vi "master_python_v3.0.vi"() -> ()   [LabVIEW 2026]
uses:
  <vilib>/Utility/error.llb/DialogType.ctl
  <vilib>/DAQmx/read.llb/DAQmx Read (Analog 1D Wfm NChan NSamp).vi
  <vilib>/DAQmx/miscellaneous.llb/DAQmx Fill In Error Info.vi
  Nanostage/Madlib.dll
  <vilib>/DAQmx/write.llb/DAQmx Write (Analog 2D DBL NChan NSamp).vi
  <vilib>/Utility/inputDevices.llb/keyboardAcquire.vi
panel:
  in  "Save Spectrum":bool
  in  "#":i32=1
  in  "Duration (s)":dbl=2.0
  out "z 2":dbl
  out "QPD":dbl
  out "Pos 0":dbl
  in  "Comment":string
  out "loop iteration":i32
  out "x start":dbl
  out "y start":dbl
  out "z start":dbl
  out "start iteration":dbl
  out "data":waveform(dbl)[](array[waveform])
  out "Numeric 2":i32
  out "Numeric":i32
  out "stop Ind":bool
  in  "Tab Control":T1(tab)
  in  "Apply Force":bool
  out "Waveform Chart 6":waveform(dbl)(graph)
  out "Waveform Chart 5":waveform(dbl)(graph)
  in  "stop":bool
  in  "Record Data":bool
  in  "New File?":bool caption="new_file"
  out "QPD Position":cluster{"Array":dbl[], "Array":dbl[]}(graph)
  out "MT channels":waveform(dbl)[](graph)
  out "QPD Precise Position":cluster{"Array":dbl[], "Array":dbl[]}(graph)
  out "QPD Sum (Volt)":waveform(dbl)(graph)
  out "x":dbl
  out "y":dbl
  out "z":dbl
  in  "<":bool
  in  ">":bool
  in  "v":bool
  in  "^":bool
  in  "Down":bool
  in  "Up":bool
  in  "Fine":dbl=50.0
  in  "Step Size (nm)":bool
  in  "Course":dbl=500.0
  in  "Enable\ntapping":bool
  in  "DELAY (ms)":u32=10
  in  "x amplitude\n(um)":dbl
  in  "speed":i32=1
  in  "z amplitude (um)":dbl
  out "# oscillations":dbl
  in  "y amplitude\n(um)":dbl min=-25.0 max=25.0 step=0.05
  in  "Samples":u16=100 min=1 step=1
  in  "Centre":bool
  in  "Power Spectrum":bool
  in  "Boolean":bool
  in  "Frequency":dbl=1.0 min=0.0 max=100.0 step=0.01
  in  "Amplitude":dbl=0.5 min=0.1 max=0.9 step=0.1
  in  "# Cycles":dbl=50.0 min=0.0 max=10000.0 step=0.001
  in  "Start Signal\nGen":bool
  in  "Desired Force (pN)":dbl step=0.01
  out "Measured Force (pN)":dbl(slide) scale=-2.0..2.0
  out "QPD nLR":waveform(dbl)(graph)
  out "QPD nBT":waveform(dbl)(graph)
  in  "Filename":path=path "C:/Users/localadmin/Desktop/220601 beadscan/7umscan2umbead.lvm"
  in  "Set 0 pN Position":bool
  out "QPD0":dbl
  in  "reinitialize?":bool
  in  "Conversion factor (pN/V)":dbl=1.0
  in  "output range":cluster{"output high":dbl, "output low":dbl}={"output high"=0.1, "output low"=-0.1} {"output low" format="%.2f"; "output high" format="%.2f"}
  in  "PID gains":T2={"proportional gain (Kc)"=0.5, "integral time (Ti, min)"=0.0, "derivative time (Td, min)"=0.0} {"derivative time (Td, min)" min=-1e-18 max=1000000000000000.0 step=1e-05 format="%.3f"; "integral time (Ti, min)" min=-1e-18 step=1e-05 format="%.6f"; "proportional gain (Kc)" min=-1e-18 step=1e-05 format="%.5f"}
  out "Setpoint":dbl
  out "PID output":dbl format="%.2f"
  # "Left= anticlockwise"
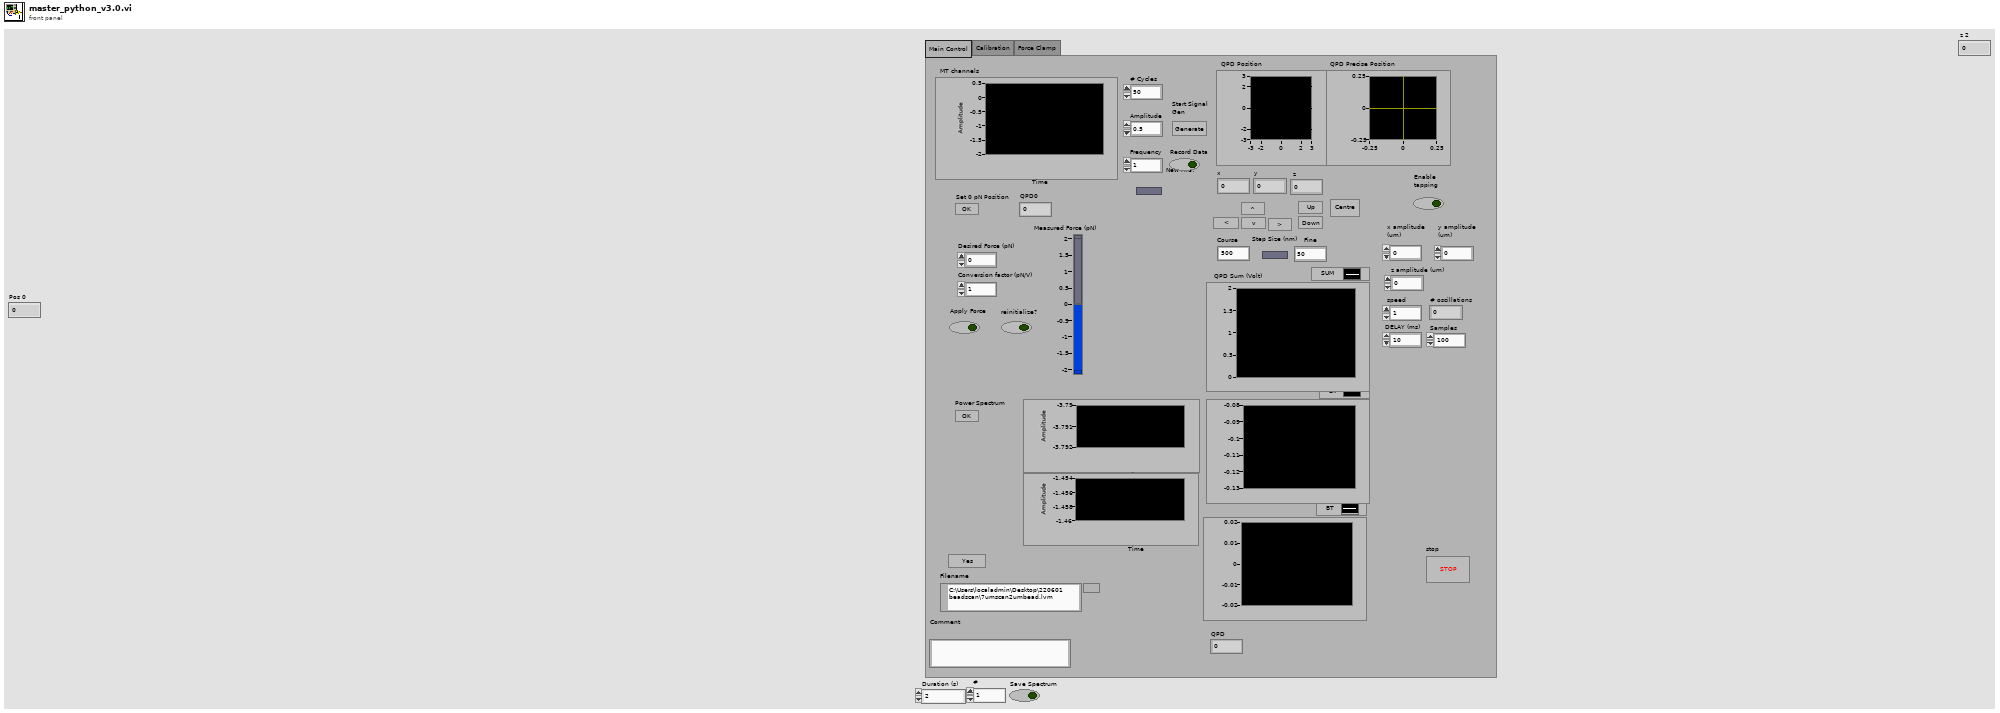
[diagram p1: front panel]
types:
  T1 = enum32{"Main Control", "Calibration", "Force Clamp"}
  T2 = cluster{"proportional gain (Kc)":dbl, "integral time (Ti, min)":dbl, "derivative time (Td, min)":dbl}
  T3 = typedef "DialogType.ctl" = u16
  T4 = enum16{"Centre", "Move", "Tapping", "Calibration"}
  T5 = cluster{"kp":dbl, "ti":dbl, "td":dbl, "index":i32, "process_variable":dbl, "derivative_action":dbl, "integrated_error":dbl, "error":dbl, "output":dbl}
  T6 = enum16{"0", "1", "2", "3", "4", "5", "6", "7", "8", "9", "A", "B", "C", "D", "E", "F", "G", "H", "I", "J", "K", "L", "M", "N", "O", "P", "Q", "R", "S", "T", "U", "V", "W", "X", "Y", "Z", "F1", "F2", "F3", "F4", "F5", "F6", "F7", "F8", "F9", "F10", "F11", "F12", "F13", "F14", "F15", "ADD", "BACK", "BACKSLASH", "CAPITAL", "COMMA", "DECIMAL", "DELETE", "DIVIDE", "DOWN", "END", "EQUALS", "ESCAPE", "GRAVE (`)", "HOME", "INSERT", "LBRACKET", "LCONTROL", "LEFT", "L ALT", "LSHIFT", "LWIN", "MINUS", "MULTIPLY", "NEXT", "NUMLOCK", "NUMPAD_0", "NUMPAD_1", "NUMPAD_2", "NUMPAD_3", "NUMPAD_4", "NUMPAD_5", "NUMPAD_6", "NUMPAD_7", "NUMPAD_8", "NUMPAD_9", "PAUSE", "PERIOD", "PRIOR (PG UP)", "RBRACKET", "RCONTROL", "RETURN", "RIGHT", "R ALT", "RSHIFT", "RWIN", "SCROLL", "SEMICOLON", "SLASH", "SPACE", "SUBTRACT", "TAB", "UP", "ENTER (num pad)", "' (quote)"}[]
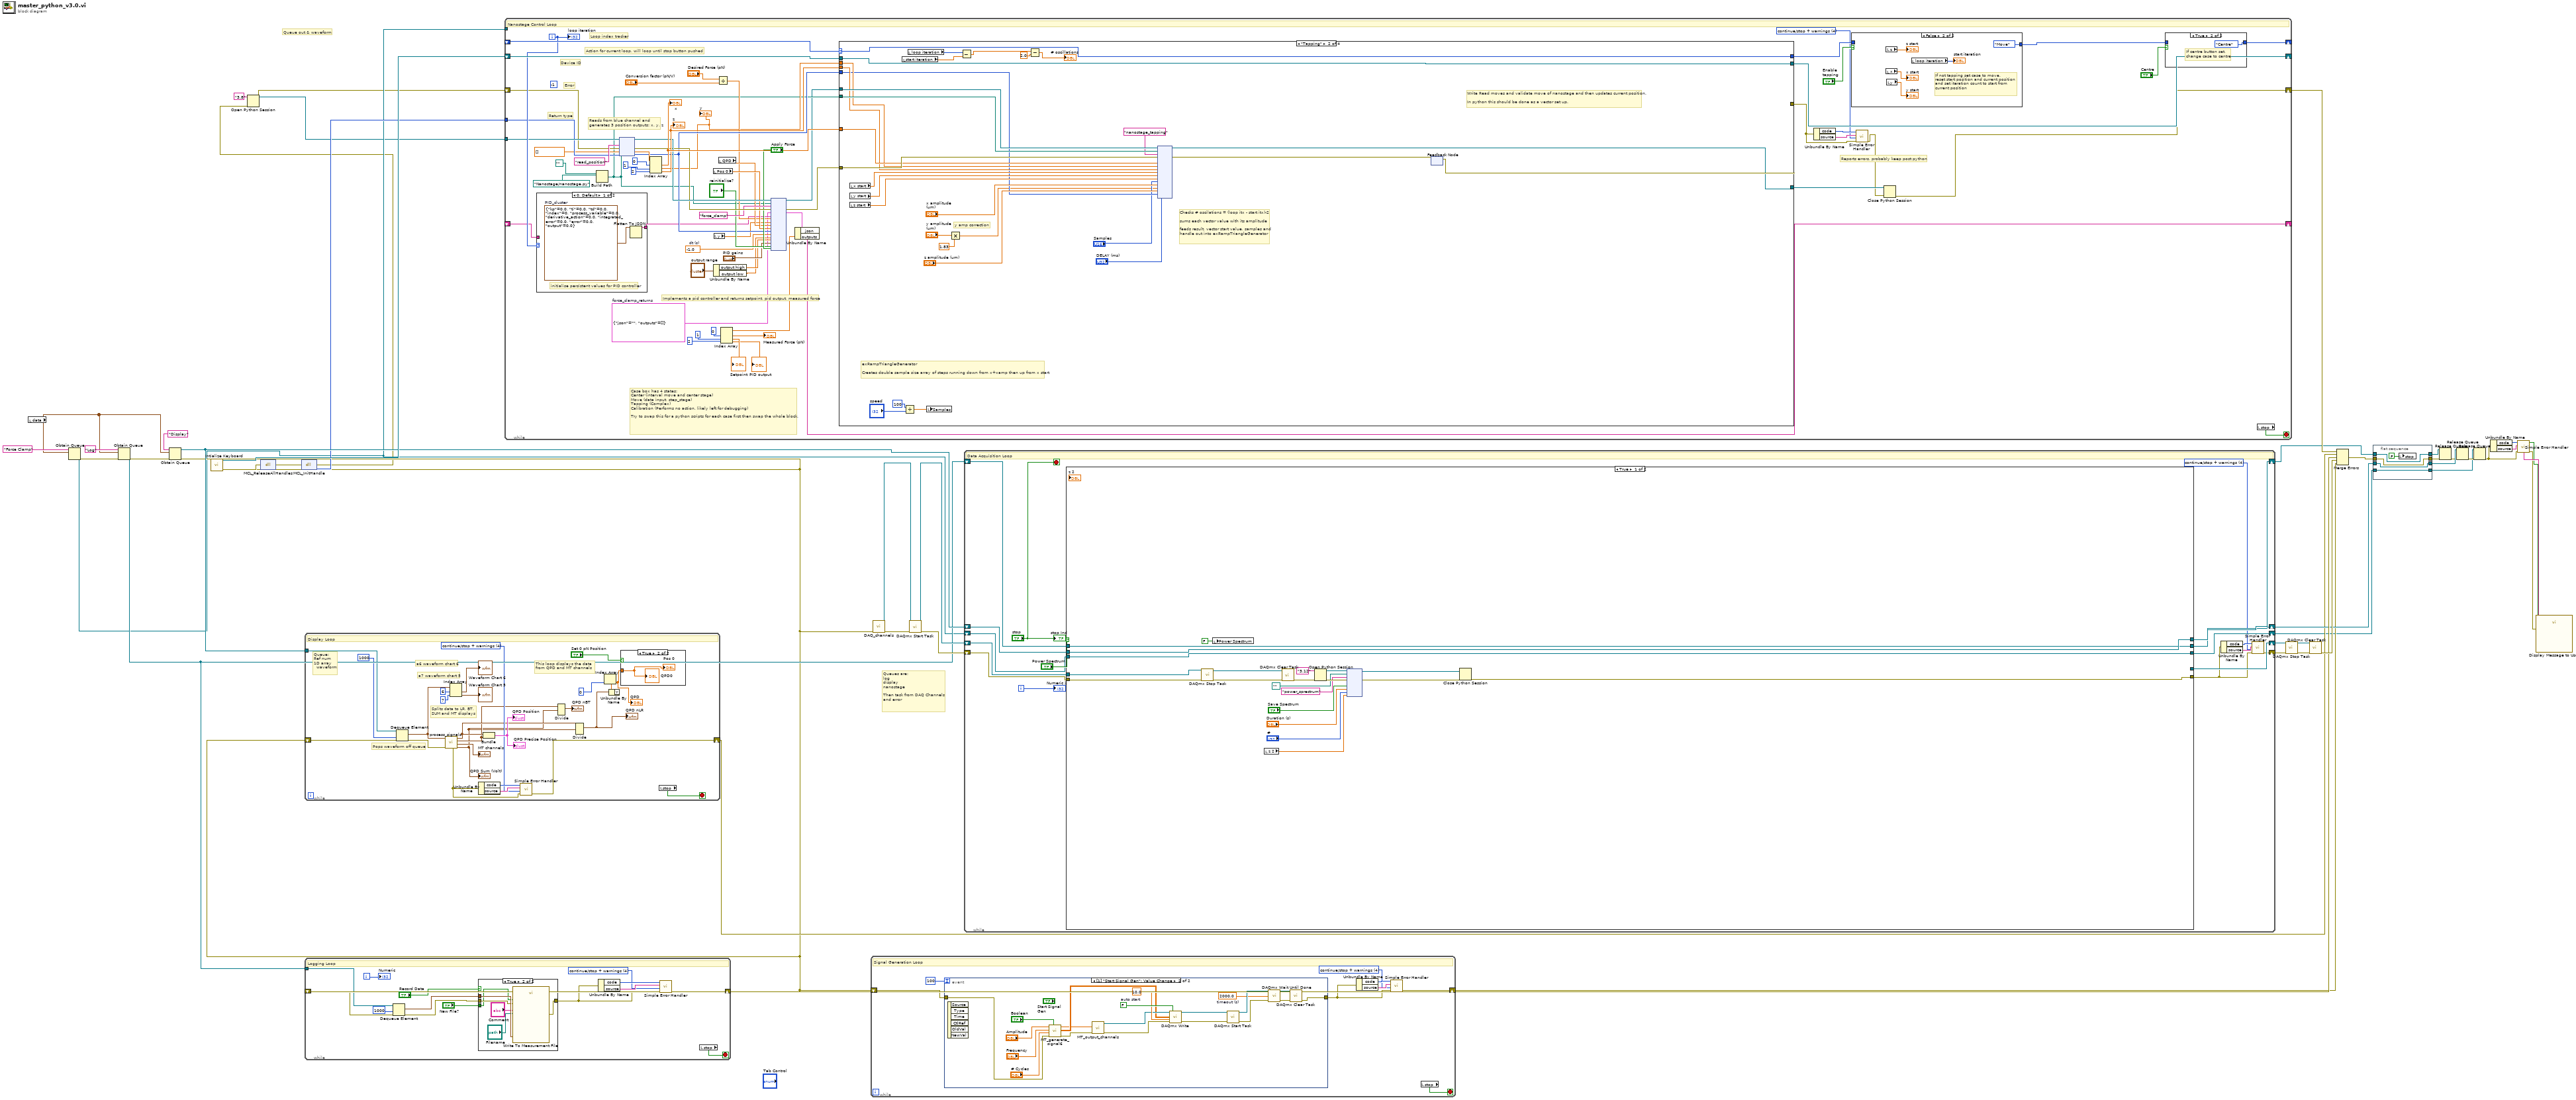
[diagram p0: block diagram]
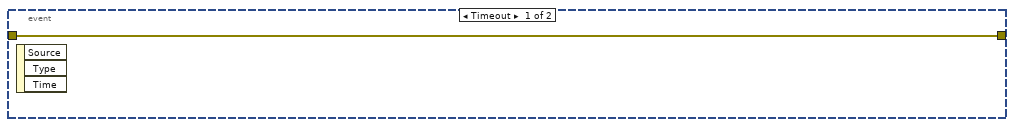
[diagram p2: hidden frame]
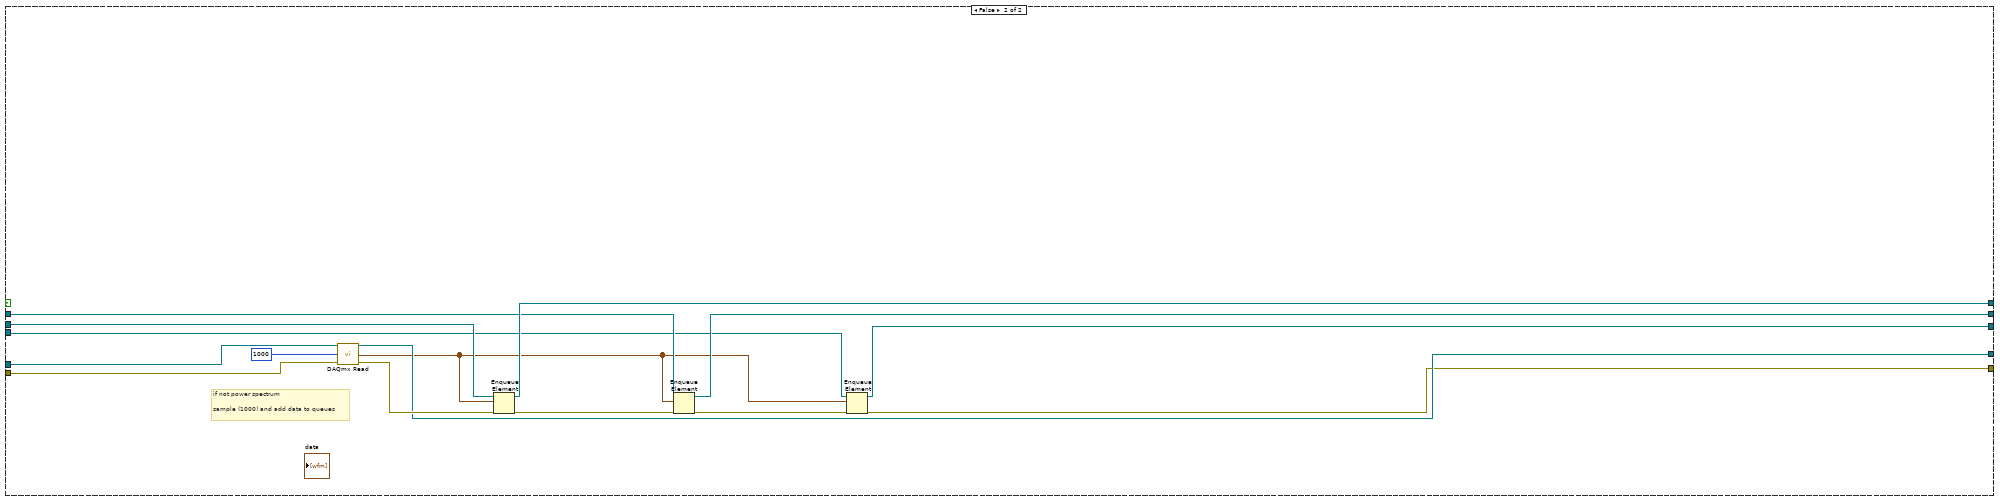
[diagram p3: hidden frame]
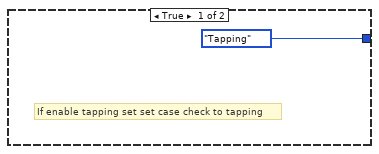
[diagram p7: hidden frame]
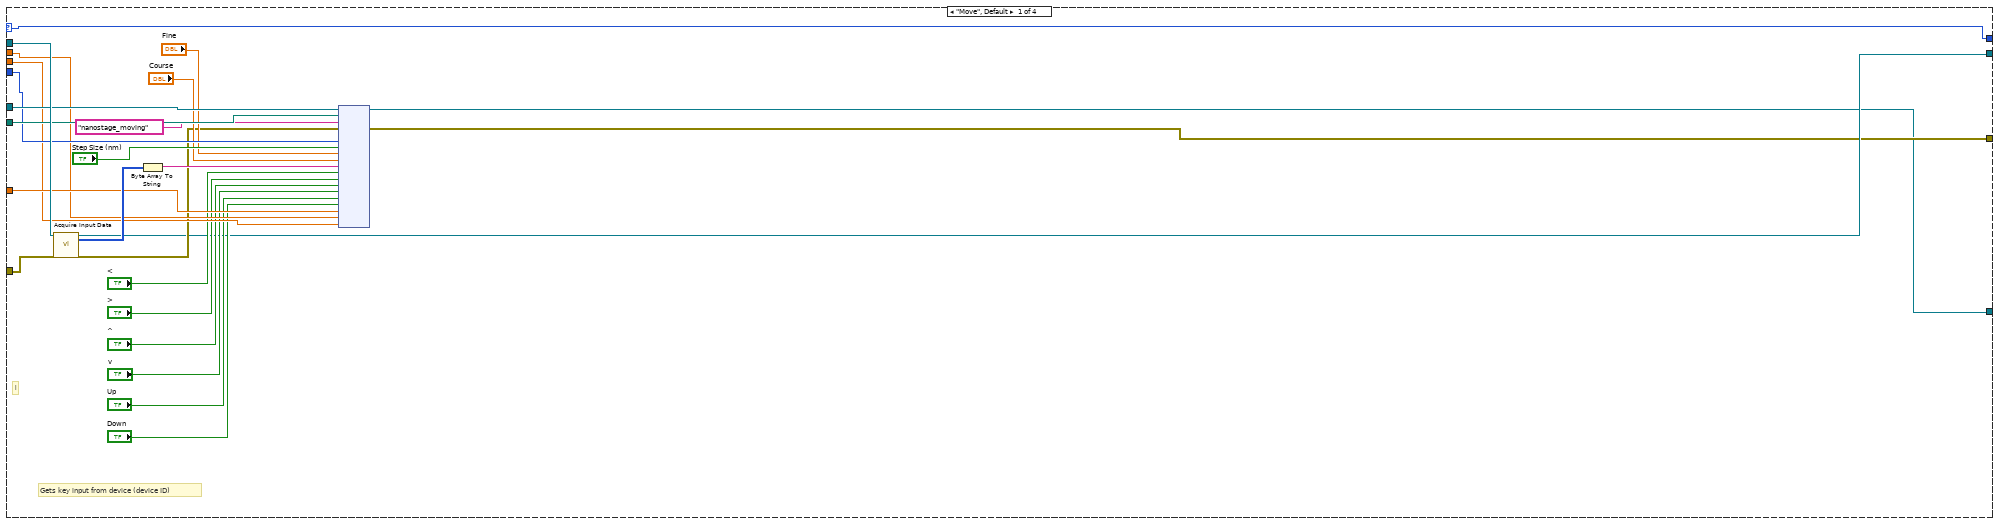
[diagram p8: hidden frame]
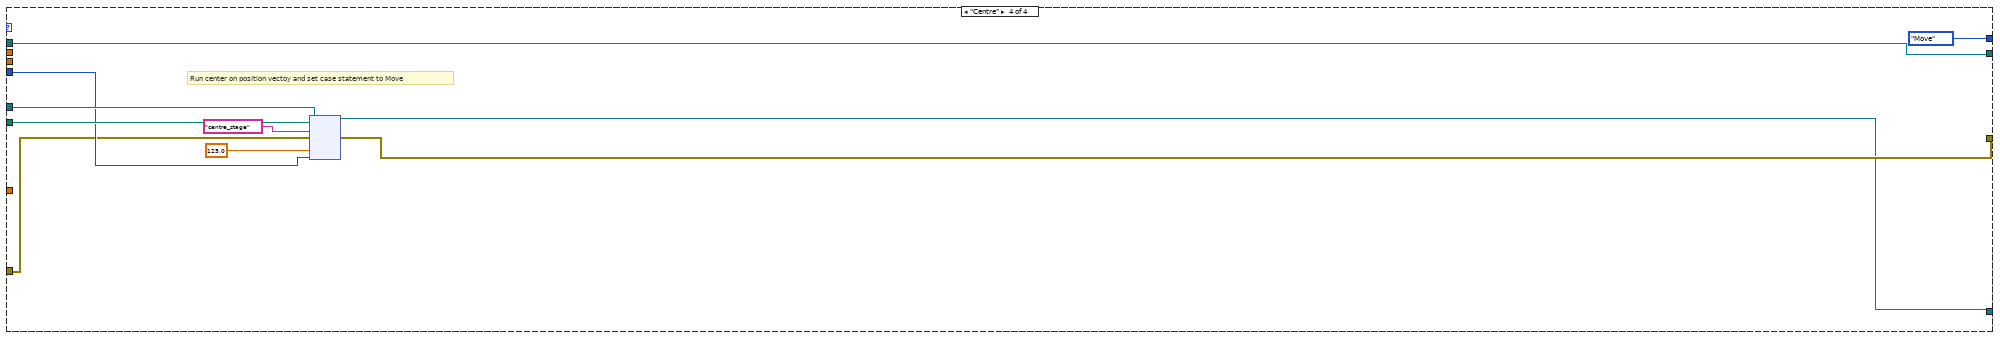
[diagram p10: hidden frame]
diagram:
  # "Queues are:\nlog\ndisplay\nnanostage\n\nThen task from DAQ Channels\nand error"
  # "Queue out & waveform"
  n1 = local read "data"() -> (w10:waveform(dbl)[])
  n2 = Obtain Queue(name (unnamed)="Force Clamp", element data type=w10) -> (queue out=w5:refnum<queue>, error out=w12:errorcluster)  [unwired: 3 in, 1 out]
  n3 = Obtain Queue(name (unnamed)="Log", element data type=w10, error in (no error)=w12) -> (queue out=w16:refnum<queue>, error out=w21:errorcluster)  [unwired: 2 in, 1 out]
  n4 = Obtain Queue(name (unnamed)="Display", element data type=w10, error in (no error)=w21) -> (queue out=w23:refnum<queue>, error out=w14:errorcluster)  [unwired: 2 in, 1 out]
  n5 = call <vilib>:"Intialize Keyboard.vi"("error in (no error)"=w14) -> ("error out"=w26:errorcluster, "device ID"=w25:refnum<k1>)  [unwired: 9 out]
  n6 = dll-call lib="C:/Users/psmr500/PycharmProjects/COMBI-Tweez/LabVIEW Microscope Control/Nanostage/MADLib.dll" fn="MCL_ReleaseAllHandles"(error in=w26) -> (error out=w27:errorcluster)  [unwired: 3 in, 1 out]
  n7 = dll-call lib="C:/Users/psmr500/PycharmProjects/COMBI-Tweez/LabVIEW Microscope Control/Nanostage/MADLib.dll" fn="MCL_InitHandle"(error in=w27) -> (error out=w2:errorcluster, "return type"=w15:i32)  [unwired: 2 in, 1 out]
  n8 = Open Python Session(python version="3.8" ("Python version"), 3:w2) -> (session out=w4:refnum<k35>, error out=w3:errorcluster)  [unwired: 1 in]
  n9 = while {
    tunnel: w23 -> [w73]
    shift-right: [w58] -> w29
    shift-left: w14 -> [w72]
    stop <- w71 stop-if-true
    w57 = T3 4 items=["no dialog", "OK message", "continue or stop message", "OK message + warnings", "continue/stop + warnings"] ("type of dialog (OK msg:1)")
    # "a7 waveform chart 5"
    # "a6 waveform chart 6"
    # "Splits data to LR, BT,\nSUM and MT displays"
    # "Pops waveform off queue"
    # "Queue:\nRef num\n1D array\n  waveform"
    # "This loop displays the data from QPD and MT channels"
    # "Display Loop"
    n10 = Dequeue Element(queue=w73, timeout in ms (-1)=1000, error in (no error)=w72) -> (element=w63:waveform(dbl)[], error out=w65:errorcluster)  [unwired: 2 out]
    n11 = call "process_signals.vi"("error in (no error)"=w65, "data"=w63) -> ("SUM"=w53:waveform(dbl), "MT"=→"MT channels":waveform(dbl)[], "BT"=w54:waveform(dbl), "LR"=w55:waveform(dbl), "error out"=w66:errorcluster)  [unwired: 5 in]
    "QPD Sum (Volt)" <- w53
    n12 = Index Array(array=w63, index #1=6 ("index"), index #2=7 ("index")) -> (element #1=→"Waveform Chart 6":waveform(dbl), element #2=→"Waveform Chart 5":waveform(dbl))
    n13 = Unbundle By Name(w66) -> ("code"=w68:i32, "source"=w67:string)
    n14 = Bundle("LR"=w55, "BT"=w54) -> (→"QPD Position" →"QPD Precise Position":cluster{"LR":waveform(dbl), "BT":waveform(dbl)})  [unwired: 1 in]
    n15 = call <vilib>:"Simple Error Handler.vi"("error code (no error:0)"=w68, "error source (\" \")"=w67, "type of dialog (OK msg:1)"=w57, "error in (no error)"=w66) -> ("error out"=w58:errorcluster)  [unwired: 1 in, 4 out]
    n16 = Divide(1:w53, 2:w54) -> (0:→"QPD nBT":waveform(dbl))  [unwired: 1 in, 1 out]
    n17 = Divide(1:w53, 2:w55) -> (0:w50:waveform(dbl))  [unwired: 1 in, 1 out]
    "QPD nLR" <- w50
    n18 = Unbundle By Name(w50) -> ("Y"=w51:dbl[])
    n19 = Index Array(array=w51, index=0) -> (element=w48:dbl)
    "QPD" <- w48
    n20 = case shown="True" "Set 0 pN Position" {
      tunnel: w48 -> [_ w74]
      frame False {
      }
      frame True {
        "Pos 0" <- w74
        "QPD0" <- w74
      }
    }
    n21 = local read "stop"() -> (w71:bool)
  }
  n22 = while {
    shift-right: [w76] -> w33
    shift-left: w14 -> [w88]
    tunnel: w16 -> [w87]
    i -> [w82]
    stop <- w77 stop-if-true
    w75 = T3 4 items=["no dialog", "OK message", "continue or stop message", "OK message + warnings", "continue/stop + warnings"] ("type of dialog (OK msg:1)")
    # "Logging Loop"
    n23 = Dequeue Element(queue=w87, timeout in ms (-1)=1000, error in (no error)=w88) -> (element=w84:waveform(dbl)[], error out=w85:errorcluster)  [unwired: 2 out]
    n24 = case shown="True" "Record Data" {
      tunnel: [w89 w95] -> w78
      tunnel: w84 -> [_ w94]
      tunnel: "New File?" -> [_ w91]
      tunnel: w85 -> [w89 w93]
      frame False {
      }
      frame True {
        n25 = call "Write To Measurement File"("Signals"=w94, "new_file"=w91, "error in (no error)"=w93, "Filename"="Filename", "Comment"="Comment") -> ("error out"=w95:errorcluster)  [unwired: 12 in, 2 out]
      }
    }
    n26 = Unbundle By Name(w78) -> ("code"=w80:i32, "source"=w79:string)
    n27 = call <vilib>:"Simple Error Handler.vi"("error code (no error:0)"=w80, "error source (\" \")"=w79, "type of dialog (OK msg:1)"=w75, "error in (no error)"=w78) -> ("error out"=w76:errorcluster)  [unwired: 1 in, 4 out]
    n28 = local read "stop"() -> (w77:bool)
    "Numeric" <- w82
  }
  n29 = while {
    shift-right: [w96] -> w24
    shift-left: w3 -> [w139]
    shift-right: [w152] -> _
    shift-left: w25 -> [w154]
    shift-right: [w148] -> _
    shift-left: _ -> [w153]
    tunnel: w15 -> [w138]
    tunnel: w5 -> [_]
    shift-right: [w111] -> _
    shift-left: _ -> [w142]
    tunnel: w4 -> [w140]
    i -> [w143]
    stop <- w158 stop-if-true
    w120 = -1.0  # dt (s)
    w113 = cluster{"json":string, "outputs":dbl[]} {"json"="", "outputs"=[]}  # force_clamp_returns
    (unwired) -1 ("timeout in ms (-1)")
    w147 = T3 4 items=["no dialog", "OK message", "continue or stop message", "OK message + warnings", "continue/stop + warnings"] ("type of dialog (OK msg:1)")
    # "Reports errors, probably keep post python"
    # "Case box has 4 states:\nCenter (interval move and center stage)\nMove (data input, step_stage)\nTapping (Complex)\nCalibration (Performs no action, likely left for debugging)\n\nTry to swap this for a python scripts for each case first then swap the whole block."
    # "Action for current loop, will loop until stop button pushed"
    # "Implements a pid controller and returns setpoint, pid output, measured force"
    # "Return type"
    # "Device ID"
    # "Error"
    # "Reads from blue channel and \ngenerates 3 position outputs: x, y, z"
    # "Loop index tracker"
    # "Nanostage Control Loop"
    n30 = case shown="0, Default" w143 {
      tunnel: [w159 w161] -> w114
      tunnel: w142 -> [_ w161]
      frame 0, Default {
        w160 = T5 {"kp"=0.0, "ti"=0.0, "td"=0.0, "index"=0, "process_variable"=0.0, "derivative_action"=0.0, "integrated_error"=0.0, "error"=0.0, "output"=0.0}  # PID_cluster
        # "initialise persistent values for PID controller"
        n31 = Flatten To JSON(anything=w160) -> (JSON string=w159:string)  [unwired: 2 in, 1 out]
      }
      frame 1 {
      }
    }
    n32 = Build Path(base path=path "", name or relative path=path "Nanostage/nanostage.py") -> (appended path=w100:path)
    n33 = node(w140, w100, "read_position" ("function name"), w139, dbl[] [], w138) -> (w130:refnum<k35>, w129:errorcluster, w136:dbl[], w119:i32)  [unwired: 2 out]
    n34 = Index Array(array=w136, index #1=0 ("index"), index #2=1 ("index"), index #3=2 ("index")) -> (element #1=w132:dbl, element #2=w101:dbl, element #3=w131:dbl)
    "x" <- w132
    "y" <- w101
    "z" <- w131
    n35 = local read "Pos 0"() -> (w118:dbl)
    n36 = Unbundle By Name("output range") -> ("output high"=w122:dbl, "output low"=w121:dbl)
    n37 = local read "y"() -> (w116:dbl)
    n38 = Divide(x="Desired Force (pN)", y="Conversion factor (pN/V)") -> (x/y=w115:dbl)
    n39 = local read "QPD"() -> (w117:dbl)
    n40 = node(w130, w100, "force_clamp" ("function name"), w129, w113, w114, w115, w116, w117, w118, w119, w120, w121, w122, "PID gains", "reinitialize?", "Apply Force") -> (w99:refnum<k35>, w128:errorcluster, w112:cluster{"json":string, "outputs":dbl[]})  [unwired: 12 in, 2 out]
    n41 = Unbundle By Name(w112) -> ("json"=w111:string, "outputs"=w110:dbl[])
    n42 = Index Array(array=w110, index #1=0 ("index"), index #2=1 ("index"), index #3=2 ("index")) -> (element #1=→"Measured Force (pN)":dbl, element #2=→"Setpoint":dbl, element #3=→"PID output":dbl)
    n43 = case shown="\"Tapping\"" w153 {
      selector: w153 -> [w192 w216 w236 _]
      tunnel: w128 -> [w193 w209 w234 w247]
      tunnel: w119 -> [w188 w198 w235 w248]
      tunnel: [w171 w210 w228 w250] -> w155
      tunnel: w132 -> [w182 w207 w238 _]
      tunnel: w101 -> [w181 w206 w237 _]
      tunnel: w131 -> [w180 w205 _ _]
      tunnel: w154 -> [w194 w217 w227 w254]
      tunnel: [w192 w216 w236 T4."Move"] -> w151
      tunnel: [w172 w217 w227 w254] -> w152
      tunnel: w100 -> [w190 w213 _ w253]
      tunnel: w99 -> [w191 w214 w226 w252]
      tunnel: [w170 w208 w226 w246] -> w98
      frame "Move", Default {
        # "Gets key input from device (device ID)"
        # "l"
        n44 = call-poly <vilib>:"Acquire Input Data.vi"("device ID"=w194, "error in (no error)"=w193) -> ("device ID"=w172:refnum<k1>, "keys pressed"=w184:T6, "error out"=w173:errorcluster)  [unwired: 15 out]
        n45 = Byte Array To String(unsigned byte array=w184) -> (string=w183:string)
        n46 = node(w191, w190, "nanostage_moving" ("function name"), w173, w188, "Step Size (nm)", "Fine", "Course", w183, "<", ">", "^", "v", "Up", "Down", w182, w181, w180) -> (w170:refnum<k35>, w171:errorcluster)  [unwired: 16 in, 2 out]
      }
      frame "Tapping" {
        # "Write Read moves and validate move of nanostage and then updates current position.\n\nIn python this should be done as a vector set up."
        # "exRampTriangleGenerator\n\nCreates double sample size array of steps running down from x+xamp then up from x start"
        # "Checks # oscilations = (loop itx - start itx)-2\n\nsums each vector value with its amplitude\n\nfeeds result, vector start value, samples and \nhandle out into exRampTriangleGenerator"
        # "y amp correction"
        n47 = local read "x start"() -> (w204:dbl)
        n48 = local read "y start"() -> (w203:dbl)
        n49 = local read "z start"() -> (w202:dbl)
        n50 = local read "start iteration"() -> (w222:dbl)
        n51 = Divide(x=100, y="speed") -> (x/y=w223:dbl)
        n52 = local read "loop iteration"() -> (w221:i32)
        n53 = local write "Samples"(w223) -> ()
        n54 = Multiply(x="y amplitude\n(um)", y=1.83) -> (x*y=w195:dbl)
        n55 = Subtract(x=w221, y=w222) -> (x-y=w220:dbl)
        n56 = Subtract(x=w220, y=2.0) -> (x-y=→"# oscillations":dbl)
        n57 = node(w214, w213, "nanostage_tapping" ("function name"), w209, w207, w206, w205, w204, w203, w202, "Samples", "x amplitude\n(um)", w195, "z amplitude (um)", w198, "DELAY (ms)") -> (w208:refnum<k35>, w211:errorcluster)  [unwired: 14 in, 2 out]
        n58 = feedback-in #1(w211) -> ()
        n59 = feedback #1() -> (w210:errorcluster)  [unwired: 1 in]
      }
      frame "Calibration" {
        n60 = flat-sequence {
          tunnel: w234 -> [w239]
          tunnel: [w239] -> w229
          tunnel: [w240] -> w230
          tunnel: w229 -> [w240]
          tunnel: w235 -> [_]
          tunnel: w238 -> [_]
          tunnel: w237 -> [_]
          tunnel: [w241] -> w231
          tunnel: w230 -> [w241]
          tunnel: [w242] -> w232
          tunnel: w231 -> [w242]
          tunnel: [w244] -> _
          tunnel: w235 -> [w244]
          tunnel: [w243] -> w233
          tunnel: w232 -> [w243]
          tunnel: w233 -> [w245]
          tunnel: [w245] -> w228
          frame #0 {
          }
          frame #1 {
          }
          frame #2 {
          }
          frame #3 {
          }
          frame #4 {
          }
          frame #5 {
          }
        }
      }
      frame "Centre" {
        # "Run center on position vectoy and set case statement to Move"
        n61 = node(w252, w253, "centre_stage" ("function name"), w247, 125.0 ("Destination"), w248) -> (w246:refnum<k35>, w250:errorcluster)  [unwired: 4 in, 2 out]
      }
    }
    n62 = Unbundle By Name(w155) -> ("code"=w157:i32, "source"=w156:string)
    n63 = case shown="False" "Enable\ntapping" {
      tunnel: w151 -> [_ _]
      tunnel: [T4."Tapping" T4."Move"] -> w146
      frame True {
        # "If enable tapping set set case check to tapping"
      }
      frame False {
        # "If not tapping set case to move.\nreset start position and current position \nand set iteration count to start from \ncurrent position"
        n64 = local read "z"() -> (→"z start":dbl)
        n65 = local read "x"() -> (→"x start":dbl)
        n66 = local read "y"() -> (→"y start":dbl)
        n67 = local read "loop iteration"() -> (→"start iteration":i32)
      }
    }
    n68 = call <vilib>:"Simple Error Handler.vi"("error code (no error:0)"=w157, "error source (\" \")"=w156, "type of dialog (OK msg:1)"=w147, "error in (no error)"=w155) -> ("error out"=w97:errorcluster)  [unwired: 1 in, 4 out]
    n69 = Close Python Session(session in=w98, error in=w97) -> (11:w96:errorcluster)
    n70 = case shown="True" "Centre" {
      tunnel: [w162 T4."Centre"] -> w148
      tunnel: w146 -> [w162 _]
      frame False {
        # "If not centre no effect"
      }
      frame True {
        # "If centre button set, \nchange case to centre"
      }
    }
    n71 = local read "stop"() -> (w158:bool)
    "loop iteration" <- w143
  }
  n72 = while {
    shift-right: [w257] -> w13
    shift-left: w14 -> [w262]
    stop <- w263 stop-if-true
    w258 = T3 4 items=["no dialog", "OK message", "continue or stop message", "OK message + warnings", "continue/stop + warnings"] ("type of dialog (OK msg:1)")
    # "Signal Generation Loop"
    n73 = event shown="[1] \"Start Signal Gen\": Value Change" {
      selector: _ -> [_ _]
      dyn-events: _ -> [_ _]
      timeout: 100 -> [_ _]
      tunnel: [w264 w267] -> w256
      tunnel: w262 -> [w264 w266]
      event Timeout {
        n74 = event-data() -> ()  [unwired: 1 in, 3 out]
      }
      event "Start Signal\nGen": Value Change {
        w276 = 2000.0  # timeout (s)
        w275 = FALSE  # auto start
        n75 = event-data() -> ()  [unwired: 1 in, 6 out]
        n76 = call "MT_generate_signal6.vi"("Direction"="Boolean", "error in (no error)"=w266, "# cycles"="# Cycles", "frequency"="Frequency", "amplitude"="Amplitude") -> ("error out"=w272:errorcluster, "signals out"=w270:dbl[][], "# samples"=w269:dbl)  [unwired: 4 in]
        n77 = call "MT_output_channels.vi"("error in"=w272, "number of samples"=w269) -> ("error out"=w271:errorcluster, "task out"=w273:refnum<k21>)  [unwired: 8 in]
        n78 = call-poly <vilib>:"DAQmx Write.vi"("task/channels in"=w273, "auto start"=w275, "data"=w270, "timeout"=10.0, "error in"=w271) -> ("task out"=w280:refnum<k21>, "error out"=w281:errorcluster)  [unwired: 8 in, 1 out]
        n79 = call <vilib>:"DAQmx Start Task.vi"("task/channels in"=w280, "error in"=w281) -> ("task out"=w277:refnum<k21>, "error out"=w278:errorcluster)  [unwired: 12 in]
        n80 = call <vilib>:"DAQmx Wait Until Done.vi"("task/channels in"=w277, "timeout (sec)"=w276, "error in"=w278) -> ("task out"=w282:refnum<k21>, "error out"=w279:errorcluster)  [unwired: 11 in]
        n81 = call <vilib>:"DAQmx Clear Task.vi"("task in"=w282, "error in"=w279) -> ("error out"=w267:errorcluster)  [unwired: 13 in]
      }
    }
    n82 = Unbundle By Name(w256) -> ("code"=w260:i32, "source"=w259:string)
    n83 = call <vilib>:"Simple Error Handler.vi"("error code (no error:0)"=w260, "error source (\" \")"=w259, "type of dialog (OK msg:1)"=w258, "error in (no error)"=w256) -> ("error out"=w257:errorcluster)  [unwired: 1 in, 4 out]
    n84 = local read "stop"() -> (w263:bool)
  }
  n85 = call "DAQ_channels.vi"("error in"=w14) -> ("error out"=w41:errorcluster, "task out"=w42:refnum<k21>)  [unwired: 9 in]
  n86 = call <vilib>:"DAQmx Start Task.vi"("task/channels in"=w42, "error in"=w41) -> ("task out"=w45:refnum<k21>, "error out"=w46:errorcluster)  [unwired: 12 in]
  n87 = while {
    shift-right: [w286] -> w40
    shift-left: w46 -> [w301]
    shift-right: [w298] -> w32
    shift-left: w23 -> [w299]
    shift-right: [w295] -> w28
    shift-left: w45 -> [w300]
    shift-right: [w290] -> w20
    shift-left: w16 -> [w289]
    shift-right: [w287] -> w6
    shift-left: w5 -> [w288]
    i -> [w296]
    stop <- "stop" stop-if-true
    w285 = T3 4 items=["no dialog", "OK message", "continue or stop message", "OK message + warnings", "continue/stop + warnings"] ("type of dialog (OK msg:1)")
    # "Data Acquisition Loop"
    n88 = case shown="True" "Power Spectrum" {
      tunnel: w301 -> [w321 w337]
      tunnel: w300 -> [w322 w335]
      tunnel: w299 -> [w320 w334]
      tunnel: [w320 w333] -> w298
      tunnel: [_ w332] -> w295
      tunnel: [w302 w326] -> w291
      tunnel: w289 -> [w319 w330]
      tunnel: [w319 w328] -> w290
      tunnel: w288 -> [w317 w325]
      tunnel: [w317 w324] -> w287
      frame True {
        n89 = call <vilib>:"DAQmx Stop Task.vi"("task/channels in"=w322, "error in"=w321) -> ("task out"=w304:refnum<k21>, "error out"=w303:errorcluster)  [unwired: 12 in]
        n90 = local write "Power Spectrum"(FALSE ("Power Spectrum")) -> ()
        n91 = local read "z 2"() -> (w307:dbl)
        n92 = call <vilib>:"DAQmx Clear Task.vi"("task in"=w304, "error in"=w303) -> ("error out"=w315:errorcluster)  [unwired: 13 in]
        n93 = Open Python Session(python version="3.12" ("Python version"), 3:w315) -> (session out=w313:refnum<k35>, error out=w314:errorcluster)  [unwired: 1 in]
        n94 = node(w313, path "" ("module path"), "power_sprectrum" ("function name"), w314, "Save Spectrum", "Duration (s)", "#", w307) -> (w306:refnum<k35>, w305:errorcluster)  [unwired: 6 in, 2 out]
        n95 = Close Python Session(session in=w306, error in=w305) -> (11:w302:errorcluster)
      }
      frame False {
        # "if not power spectrum\n\nsample (1000) and add data to queues"
        n96 = call-poly <vilib>:"DAQmx Read.vi"("task/channels in"=w335, "number of samples per channel"=1000, "error in"=w337) -> ("task out"=w332:refnum<k21>, "data"=w323:waveform(dbl)[], "error out"=w336:errorcluster)  [unwired: 10 in]
        n97 = Enqueue Element(queue=w334, element=w323, error in (no error)=w336) -> (queue out=w333:refnum<queue>, error out=w329:errorcluster)  [unwired: 2 out]
        n98 = Enqueue Element(queue=w330, element=w323, error in (no error)=w329) -> (queue out=w328:refnum<queue>, error out=w327:errorcluster)  [unwired: 2 out]
        n99 = Enqueue Element(queue=w325, element=w323, error in (no error)=w327) -> (queue out=w324:refnum<queue>, error out=w326:errorcluster)  [unwired: 2 out]
      }
    }
    n100 = Unbundle By Name(w291) -> ("code"=w293:i32, "source"=w292:string)
    n101 = call <vilib>:"Simple Error Handler.vi"("error code (no error:0)"=w293, "error source (\" \")"=w292, "type of dialog (OK msg:1)"=w285, "error in (no error)"=w291) -> ("error out"=w286:errorcluster)  [unwired: 1 in, 4 out]
    "Numeric 2" <- w296
    "stop Ind" <- "stop"
  }
  n102 = call <vilib>:"DAQmx Stop Task.vi"("task/channels in"=w28, "error in"=w40) -> ("task out"=w38:refnum<k21>, "error out"=w39:errorcluster)  [unwired: 12 in]
  n103 = call <vilib>:"DAQmx Clear Task.vi"("task in"=w38, "error in"=w39) -> ("error out"=w34:errorcluster)  [unwired: 13 in]
  n104 = Merge Errors(w24, w29, w33, w34, w13) -> (w30:errorcluster)
  n105 = flat-sequence {
    tunnel: w32 -> [w342]
    tunnel: [w342] -> w31
    tunnel: w30 -> [w341]
    tunnel: [w341] -> w18
    tunnel: w20 -> [w339]
    tunnel: [w339] -> w19
    tunnel: [w338] -> w7
    tunnel: w6 -> [w338]
    frame #0 {
      n106 = local write "stop"(FALSE ("create if not found? (T)")) -> ()
    }
  }
  n107 = Release Queue(queue=w19, error in (no error)=w18) -> (error out=w17:errorcluster)  [unwired: 1 in, 2 out]
  n108 = Release Queue(queue=w31, error in (no error)=w17) -> (error out=w9:errorcluster)  [unwired: 1 in, 2 out]
  n109 = Release Queue(queue=w7, error in (no error)=w9) -> (error out=w8:errorcluster)  [unwired: 1 in, 2 out]
  n110 = Unbundle By Name(w8) -> ("code"=w44:i32, "source"=w43:string)
  n111 = call <vilib>:"Simple Error Handler.vi"("error code (no error:0)"=w44, "error source (\" \")"=w43, "error in (no error)"=w8) -> ("error?"=w35:bool, "error out"=w36:errorcluster, "message"=w37:string)  [unwired: 2 in, 2 out]
  n112 = call "Display Message to User"("error in (no error)"=w36, "Enable"=w35, "Message"=w37) -> ()  [unwired: 7 in, 2 out]
